vi "总磷总氮量程读取.vi"(8 "error in (no error)":errorcluster caption="错误输入（无错误）", 11 "测量参数":enum16{"COD", "氨氮", "总氮", "总磷"}(ring)) -> (0 "error out":errorcluster caption="错误输出", 3 "量程参数读取":T1)   [LabVIEW 2016, in "斯坦道总磷总氮.lvlib"]
panel:
  out "第二个子数组":u16[](array[numeric]) format="%4x"
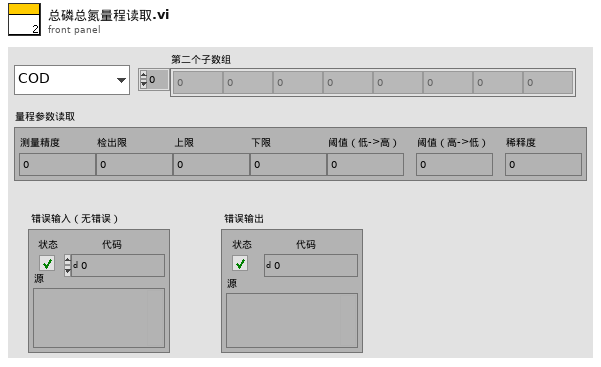
[diagram p1: front panel]
types:
  T1 = cluster{"测量精度":u16, "检出限":dbl, "上限":dbl, "下限":dbl, "阈值（低->高）":dbl, "阈值（高->低）":dbl, "稀释度":dbl}
  T2 = cluster{"FLOAT[0]":sgl, "FLOAT[1]":sgl, "FLOAT[2]":sgl, "FLOAT[3]":sgl, "FLOAT[4]":sgl}
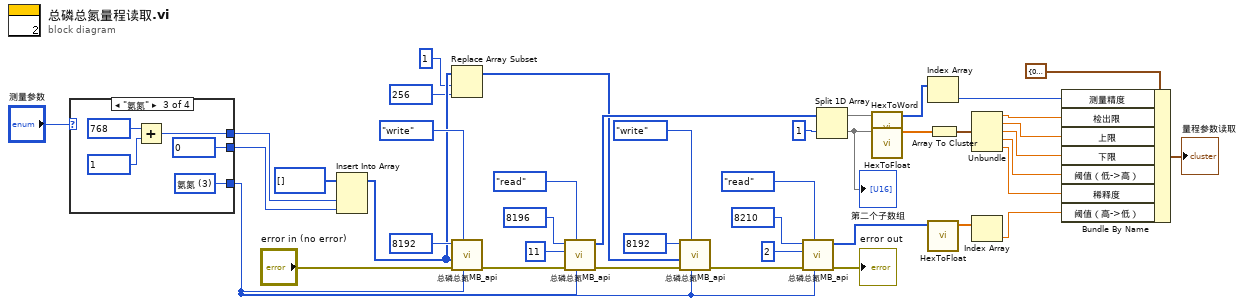
[diagram p0: block diagram]
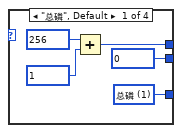
[diagram p2: hidden frame]
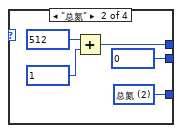
[diagram p3: hidden frame]
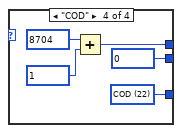
[diagram p4: hidden frame]
diagram:
  n1 = case shown="\"氨氮\"" "测量参数" {
    tunnel: [w43 w52 w57 w62] -> w12
    tunnel: [w44 w48 w53 w58] -> w37
    tunnel: [u16 0 ("starting address") u16 0 ("starting address") u16 0 ("starting address") u16 0 ("starting address")] -> w36
    frame "总磷", Default {
      w43 = u16 1 items=["总磷"=1, "总氮"=2, "氨氮"=3] ("站号")
      n2 = Add(x=u16 256 ("starting address"), y=u16 1 ("starting address")) -> (x+y=w44:u16)
    }
    frame "总氮" {
      w52 = u16 2 items=["总磷"=1, "总氮"=2, "氨氮"=3] ("站号")
      n3 = Add(x=u16 512 ("starting address"), y=u16 1 ("starting address")) -> (x+y=w48:u16)
    }
    frame "氨氮" {
      w57 = u16 3 items=["总磷"=1, "总氮"=2, "氨氮"=3] ("站号")
      n4 = Add(x=u16 768 ("starting address"), y=u16 1 ("starting address")) -> (x+y=w53:u16)
    }
    frame "COD" {
      w62 = u16 22 items=["总磷"=1, "总氮"=2, "氨氮"=3, "COD"=22] ("站号")
      n5 = Add(x=u16 8704 ("starting address"), y=u16 1 ("starting address")) -> (x+y=w58:u16)
    }
  }
  n6 = Insert Into Array(array=u16[] [] ("数组"), new element #1=w37, new element #2=w36) -> (w9:u16[])  [unwired: 1 in]
  n7 = Replace Array Subset(array=w9, new element=u16 256 ("starting address"), index=1 ("索引")) -> (w7:u16[])
  n8 = call "总磷总氮MB_api.vi"("Slave ID"=w12, "STEP"=enum16{"open", "read", "write", "close"}."write", "Error in"="error in (no error)", "values"=w9, "starting address"=u16 8192) -> ("error out"=w33:errorcluster)  [unwired: 4 in, 2 out]
  n9 = call "总磷总氮MB_api.vi"("Slave ID"=w12, "STEP"=enum16{"open", "read", "write", "close"}."read", "Error in"=w33, "quantity"=u16 11, "starting address"=u16 8196) -> ("error out"=w20:errorcluster, "Registers"=w30:u16[])  [unwired: 4 in, 1 out]
  n10 = call "总磷总氮MB_api.vi"("Slave ID"=w12, "STEP"=enum16{"open", "read", "write", "close"}."write", "Error in"=w20, "values"=w7, "starting address"=u16 8192) -> ("error out"=w19:errorcluster)  [unwired: 4 in, 2 out]
  n11 = call "总磷总氮MB_api.vi"("Slave ID"=w12, "STEP"=enum16{"open", "read", "write", "close"}."read", "Error in"=w19, "quantity"=u16 2, "starting address"=u16 8210) -> ("error out"=→"error out":errorcluster, "Registers"=w11:u16[])  [unwired: 4 in, 1 out]
  n12 = Split 1D Array(array=w30, index=1 ("长度")) -> (first subarray=w6:u16[], second subarray=w5:u16[])
  "第二个子数组" <- w5
  n13 = call "HexToWord.vi"("数组"=w6) -> ("WORD"=w28:u16[])  [unwired: 10 in]
  n14 = call "HexToFloat.vi"("数组"=w5) -> ("FLOAT"=w40:sgl[])  [unwired: 10 in]
  n15 = Index Array(array=w28) -> (element=w27:u16)  [unwired: 1 in]
  n16 = call "HexToFloat.vi"("数组"=w11) -> ("FLOAT"=w10:sgl[])  [unwired: 10 in]
  n17 = Array To Cluster(array=w40) -> (cluster=w26:T2)
  n18 = Unbundle(w26) -> ("FLOAT[0]"=w25:sgl, "FLOAT[1]"=w24:sgl, "FLOAT[2]"=w23:sgl, "FLOAT[3]"=w22:sgl, "FLOAT[4]"=w21:sgl)
  n19 = Index Array(array=w10) -> (element=w2:sgl)  [unwired: 1 in]
  n20 = Bundle By Name(cluster=T1 {"测量精度"=0, "检出限"=0.0, "上限"=0.0, "下限"=0.0, "阈值（低->高）"=0.0, "阈值（高->低）"=0.0, "稀释度"=0.0} ("量程参数读取"), "测量精度"=w27, "检出限"=w25, "上限"=w24, "下限"=w23, "阈值（低->高）"=w22, "稀释度"=w21, "阈值（高->低）"=w2) -> (→"量程参数读取":T1)
